vi "DataFinder_ReadFromMeasurementFile.vi"() -> ()   [LabVIEW 2023]
doc: "This example executes a text search in TDM files, TDMS files, and LVM files. The example uses the DataFinder \"Search Text\" VI for the search. The example then uses the \"Read From Measurement File\" VI to load the mass data of the search results and graphically displays the search results."
uses:
  <vilib>/userdefined/High Color/DFDataFinder.ctl
  <vilib>/DataFinder/Close Reference (Results).vi
  <vilib>/DataFinder/Close Reference (DataFinder).vi
  <vilib>/DataFinder/NI_DataFinder.lvlib
  <vilib>/userdefined/NI_DataFinder Controls.lvlib
panel:
  in  "DataFinder":T1
  out "Results Count":i32 min=0 max=0
  out "Result Signals":dynamicdata(graph)
  in  "Search Text":string="Chris"
  # "Overview: Searches for a specific text in TDM files, TDMS files, and LVM files and uses the \"Read From Measurement File\" VI to display the search results.\nRequirements: Select a registered DataFinder which has indexed the TDM Server Demo Data and has optimized the custom properties.\nInstructions:\n1. Ensure that the selected DataFinder is already running.\n2. Specify a value for Search Text.\nTo use the predefined search value ensure the folder [all users]\\Documents\\National Instruments\\DataFinder or one of its parent folders is included in your search areas.\n3. Run the VI.\n4. View the Resulting Signals."
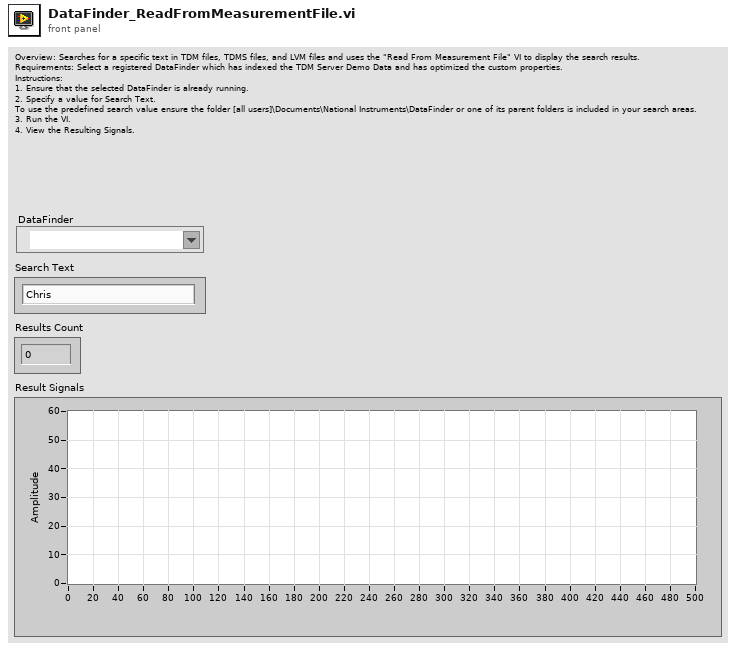
[diagram p1: front panel]
types:
  T1 = typedef "NI_DataFinder Controls.lvlib/DFDataFinder.ctl" = refnum<k21>
  T2 = typedef "NI_DataFinder Controls.lvlib/DFSearchResult.ctl" = refnum<k20>
  T3 = typedef "NI_DataFinder.lvlib/results elements.ctl" = cluster{"fullpaths":path[], "DataPlugin names":string[], "channel group names":string[], "channel names":string[]}
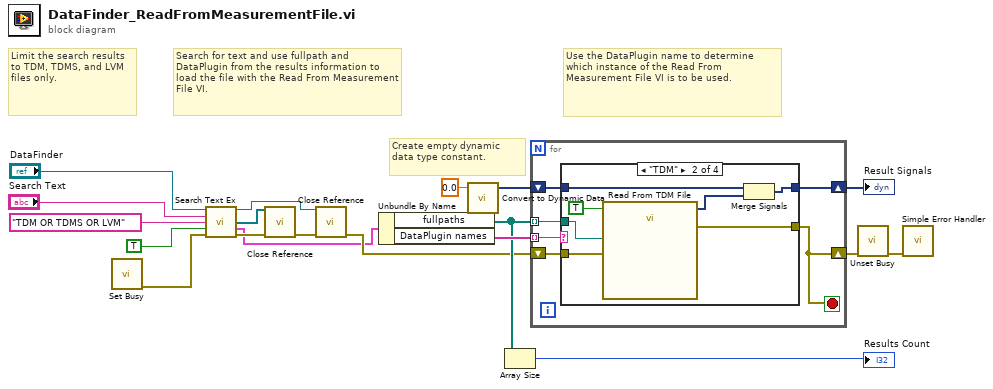
[diagram p0: block diagram]
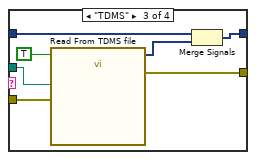
[diagram p3: hidden frame]
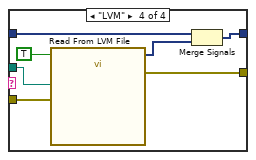
[diagram p4: hidden frame]
diagram:
  # "Create empty dynamic data type constant."
  # "Use the DataPlugin name to determine which instance of the Read From Measurement File VI is to be used."
  # "Limit the search results to TDM, TDMS, and LVM files only."
  # "Search for text and use fullpath and DataPlugin from the results information to load the file with the Read From Measurement File VI."
  n1 = call <vilib>:"Set Busy.vi"() -> ("error out"=w4:errorcluster)  [unwired: 10 in, 1 out]
  n2 = call <vilib>:"Search Text Ex.vi"("DataFinder reference"="DataFinder", "search text"="Search Text", "DataPlugin name"="TDM OR TDMS OR LVM", "fill results elements? (F)"=TRUE, "error in (no error)"=w4) -> ("DataFinder reference out"=w9:T1, "result references out"=w10:T2[], "results elements"=w5:T3, "error out"=w8:errorcluster)  [unwired: 6 in, 1 out]
  n3 = call-poly <vilib>:"Close Reference.vi"("result references"=w10, "error in (no error)"=w8) -> ("error out"=w7:errorcluster)  [unwired: 13 in]
  n4 = call-poly <vilib>:"Close Reference.vi"("DataFinder reference"=w9, "error in (no error)"=w7) -> ("error out"=w6:errorcluster)  [unwired: 13 in]
  n5 = Unbundle By Name(w5) -> ("fullpaths"=w15:path[], "DataPlugin names"=w17:string[])
  n6 = call "Convert to Dynamic Data"("Double"=0.0) -> ("Dynamic Data Type"=w11:dynamicdata)  [unwired: 3 out]
  n7 = Array Size(array=w15) -> (size(s)=→"Results Count":i32)
  n8 = for {
    shift-right: [w23] -> w16
    shift-left: w11 -> [w24]
    shift-right: [w20] -> w3
    shift-left: w6 -> [w25]
    tunnel: w17 -> [w22] mode=indexing
    tunnel: w15 -> [w21] mode=indexing
    stop <- w20 stop-if-true
    n9 = case shown="\"TDM\"" w22 {
      tunnel: w25 -> [w26 w34 w41 w48]
      tunnel: [w27 w33 w40 w47] -> w23
      tunnel: [w26 w32 w39 w46] -> w20
      tunnel: w24 -> [w27 w31 w38 w45]
      tunnel: w21 -> [_ w28 w35 w42]
      frame "", Default {
      }
      frame "TDM" {
        n10 = call "Read From TDM File"("error in (no error)"=w34, "File Name"=w28, "Reopen File"=TRUE) -> ("error out"=w32:errorcluster, "Signals"=w30:dynamicdata)  [unwired: 1 in, 6 out]
        n11 = Merge Signals(w31, w30) -> (w33:dynamicdata)
      }
      frame "TDMS" {
        n12 = call "Read From TDMS file"("error in (no error)"=w41, "File Name"=w35, "Reopen File"=TRUE) -> ("error out"=w39:errorcluster, "Signals"=w37:dynamicdata)  [unwired: 1 in, 6 out]
        n13 = Merge Signals(w38, w37) -> (w40:dynamicdata)
      }
      frame "LVM" {
        n14 = call "Read From LVM File"("error in (no error)"=w48, "File Name"=w42, "Reopen File"=TRUE) -> ("error out"=w46:errorcluster, "Signals"=w44:dynamicdata)  [unwired: 1 in, 6 out]
        n15 = Merge Signals(w45, w44) -> (w47:dynamicdata)
      }
    }
  }
  "Result Signals" <- w16
  n16 = call <vilib>:"Unset Busy.vi"("error in (no error)"=w3) -> ("error out"=w2:errorcluster)  [unwired: 10 in]
  n17 = call <vilib>:"Simple Error Handler.vi"("error in (no error)"=w2) -> ()  [unwired: 4 in, 5 out]
